vi "Postfix.vi"(8 "error in (no error)":errorcluster, 11 "Tokens":T1[](array[typedef])) -> (0 "error out":errorcluster, 3 "Postfix":T1[](array[typedef]))   [LabVIEW 2022 SP3, in "Pipes.lvlib"]
uses:
  Pipes.lvlib
  Controls/Token.ctl
  Controls/Token Type.ctl
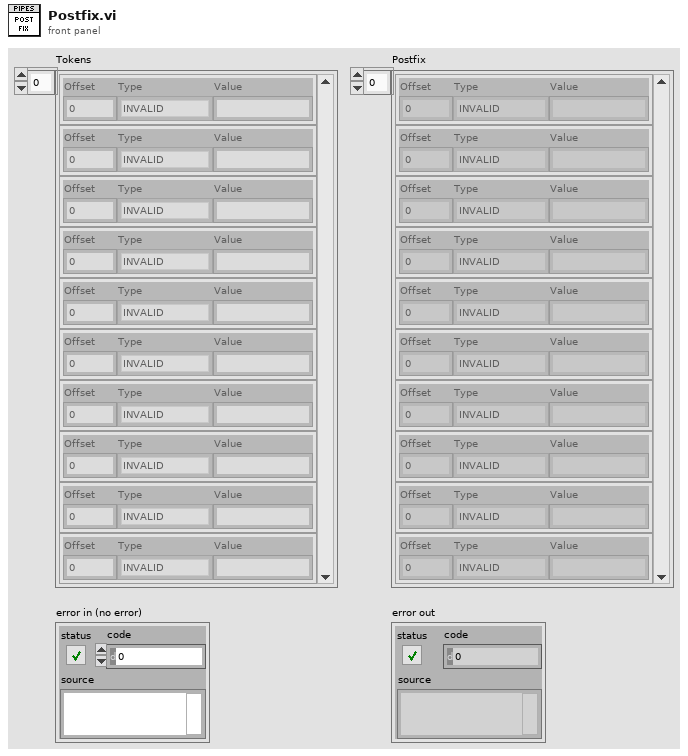
[diagram p1: front panel]
types:
  T1 = typedef "Pipes.lvlib/Token.ctl" = cluster{"Offset":i32, "Type":T2, "Value":string}
  T2 = typedef "Pipes.lvlib/Token Type.ctl" = enum8{"INVALID", "NOT", "AND", "OR", "EE", "NE", "LT", "GT", "LTE", "GTE", "PLUS", "MINUS", "MULTIPLY", "DIVIDE", "MODULUS", "LPAREN", "RPAREN", "LITERAL", "IDENTIFIER", "DEFINITION"}
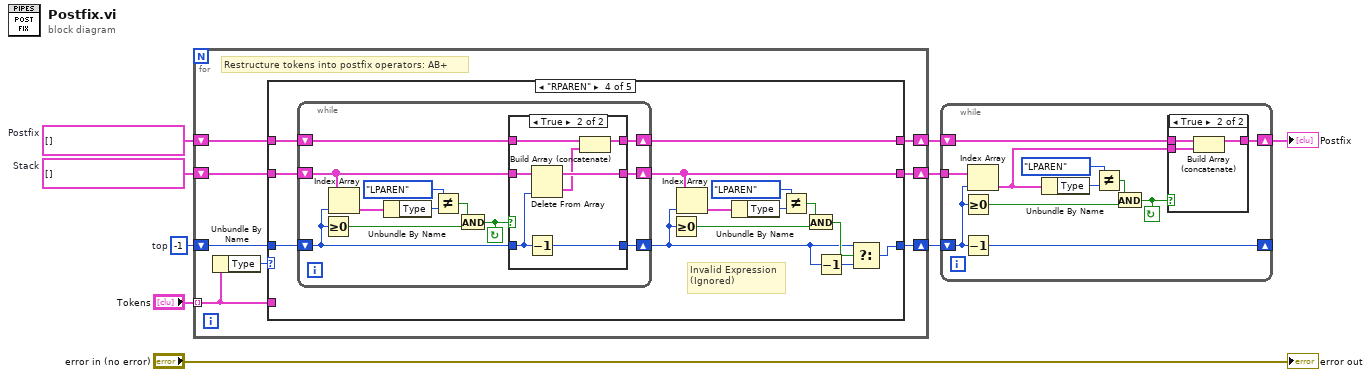
[diagram p0: block diagram]
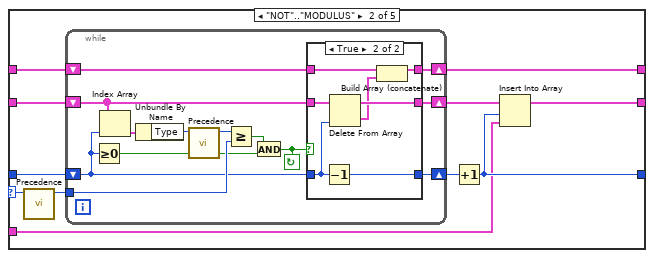
[diagram p3: hidden frame]
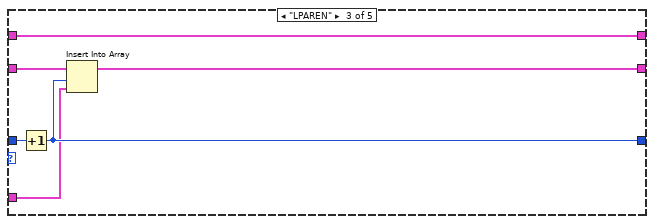
[diagram p5: hidden frame]
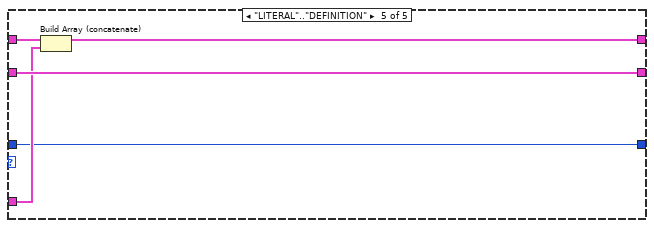
[diagram p7: hidden frame]
diagram:
  w6 = -1  # top
  w7 = T1[] []  # Stack
  w9 = T1[] []  # Postfix
  n1 = for {
    shift-right: [w16] -> w4
    shift-left: w9 -> [w15]
    tunnel: "Tokens" -> [w14] mode=indexing
    shift-right: [w12] -> w3
    shift-left: w7 -> [w13]
    shift-right: [w10] -> w1
    shift-left: w6 -> [w11]
    # "Restructure tokens into postfix operators: AB+"
    n2 = Unbundle By Name(w14) -> ("Type"=w17:T2)
    n3 = case shown="\"RPAREN\"" w17 {
      selector: w17 -> [_ w31 _ _ _]
      tunnel: [w20 w28 w60 w71 w100] -> w16
      tunnel: w15 -> [w20 w29 w60 w72 w99]
      tunnel: w14 -> [_ w21 w55 _ w98]
      tunnel: [w19 w23 w58 w66 w101] -> w12
      tunnel: w13 -> [w19 w30 w57 w74 w101]
      tunnel: w11 -> [w18 w27 w59 w73 w97]
      tunnel: [w18 w22 w56 w61 w97] -> w10
      frame "INVALID" {
      }
      frame "NOT".."MODULUS" {
        n4 = call "Precedence.vi"("Token Type"=w31) -> ("Precedence"=w26:u8)  [unwired: 10 in]
        n5 = while {
          shift-right: [w39] -> w24
          shift-left: w30 -> [w42]
          shift-right: [w40] -> w28
          shift-left: w29 -> [w41]
          tunnel: w26 -> [w37]
          shift-right: [w33] -> w25
          shift-left: w27 -> [w34]
          stop <- w32 continue-if-true
          n6 = Greater Or Equal To 0?(x=w34) -> (x >= 0?=w35:bool)
          n7 = Index Array(array=w42, index=w34) -> (element=w43:T1)
          n8 = Unbundle By Name(w43) -> ("Type"=w44:T2)
          n9 = call "Precedence.vi"("Token Type"=w44) -> ("Precedence"=w38:u8)  [unwired: 10 in]
          n10 = Greater Or Equal?(x=w38, y=w37) -> (x >= y?=w36:bool)
          n11 = And(x=w36, y=w35) -> (x .and. y?=w32:bool)
          n12 = case shown="True" w32 {
            tunnel: w42 -> [w46 w54]
            tunnel: w41 -> [w47 w50]
            tunnel: [w47 w49] -> w40
            tunnel: [w46 w53] -> w39
            tunnel: w34 -> [w45 w52]
            tunnel: [w45 w51] -> w33
            frame False {
            }
            frame True {
              n13 = Decrement(x=w52) -> (x-1=w51:i32)
              n14 = Delete From Array(array=w54, index=w52) -> (deleted portion=w48:T1, array with subset deleted=w53:T1[])  [unwired: 1 in]
              n15 = Build Array (concatenate)(w50, w48) -> (w49:T1[])
            }
          }
        }
        n16 = Increment(x=w25) -> (x+1=w22:i32)
        n17 = Insert Into Array(array=w24, index=w22, new element=w21) -> (w23:T1[])
      }
      frame "LPAREN" {
        n18 = Increment(x=w59) -> (x+1=w56:i32)
        n19 = Insert Into Array(array=w57, index=w56, new element=w55) -> (w58:T1[])
      }
      frame "RPAREN" {
        # "Invalid Expression\n(Ignored)"
        n20 = while {
          shift-right: [w86] -> w66
          shift-left: w74 -> [w85]
          shift-right: [w83] -> w71
          shift-left: w72 -> [w82]
          shift-right: [w77] -> w63
          shift-left: w73 -> [w76]
          stop <- w75 continue-if-true
          n21 = Greater Or Equal To 0?(x=w76) -> (x >= 0?=w79:bool)
          n22 = Index Array(array=w85, index=w76) -> (element=w84:T1)
          n23 = Unbundle By Name(w84) -> ("Type"=w81:T2)
          n24 = Not Equal?(x=Token_Type."LPAREN", y=w81) -> (x != y?=w78:bool)
          n25 = And(x=w78, y=w79) -> (x .and. y?=w75:bool)
          n26 = case shown="True" w75 {
            tunnel: [w88 w96] -> w86
            tunnel: w85 -> [w88 w95]
            tunnel: [w87 w94] -> w83
            tunnel: w82 -> [w87 w93]
            tunnel: [w89 w91] -> w77
            tunnel: w76 -> [w89 w90]
            frame False {
            }
            frame True {
              n27 = Decrement(x=w90) -> (x-1=w91:i32)
              n28 = Delete From Array(array=w95, index=w90) -> (deleted portion=w92:T1, array with subset deleted=w96:T1[])  [unwired: 1 in]
              n29 = Build Array (concatenate)(w93, w92) -> (w94:T1[])
            }
          }
        }
        n30 = Greater Or Equal To 0?(x=w63) -> (x >= 0?=w69:bool)
        n31 = Index Array(array=w66, index=w63) -> (element=w67:T1)
        n32 = Unbundle By Name(w67) -> ("Type"=w68:T2)
        n33 = Not Equal?(x=Token_Type."LPAREN", y=w68) -> (x != y?=w70:bool)
        n34 = And(x=w70, y=w69) -> (x .and. y?=w64:bool)
        n35 = Decrement(x=w63) -> (x-1=w62:i32)
        n36 = Select(t=w63, s=w64, f=w62) -> (s? t:f=w61:i32)
      }
      frame "LITERAL".."DEFINITION" {
        n37 = Build Array (concatenate)(w99, w98) -> (w100:T1[])
      }
    }
  }
  n38 = while {
    tunnel: w3 -> [w108]
    shift-right: [w103] -> _
    shift-left: w1 -> [w104]
    shift-right: [w112] -> w2
    shift-left: w4 -> [w111]
    stop <- w105 continue-if-true
    n39 = Greater Or Equal To 0?(x=w104) -> (x >= 0?=w106:bool)
    n40 = Decrement(x=w104) -> (x-1=w103:i32)
    n41 = Index Array(array=w108, index=w104) -> (element=w102:T1)
    n42 = Unbundle By Name(w102) -> ("Type"=w110:T2)
    n43 = Not Equal?(x=Token_Type."LPAREN", y=w110) -> (x != y?=w107:bool)
    n44 = And(x=w107, y=w106) -> (x .and. y?=w105:bool)
    n45 = case shown="True" w105 {
      tunnel: [w113 w116] -> w112
      tunnel: w111 -> [w113 w115]
      tunnel: w102 -> [_ w114]
      frame False {
      }
      frame True {
        n46 = Build Array (concatenate)(w115, w114) -> (w116:T1[])
      }
    }
  }
  "Postfix" <- w2
  "error out" <- "error in (no error)"
